vi "Set default remote state.vi"(8 "error in (no error)":errorcluster, 10 "Default remote state (Local)":u16(ring) items=["Local", "Remote"], 11 "VISA resource name":refnum<visa-resource-name>) -> (0 "error out":errorcluster, 3 "VISA resource name out":refnum<visa-resource-name>)   [LabVIEW 2020, in "Datron D4xxx.lvlib"]
doc: "This function does not affect GPIB REN state, it just sets its default value to which REN line is set after any command from this library or if you use \"Set remote state\" VI with default parameter."
uses:
  Datron D4xxx.lvlib
  Private/vars.vi
panel:
  out "VISA ID":i32
  # "Just some work variables"
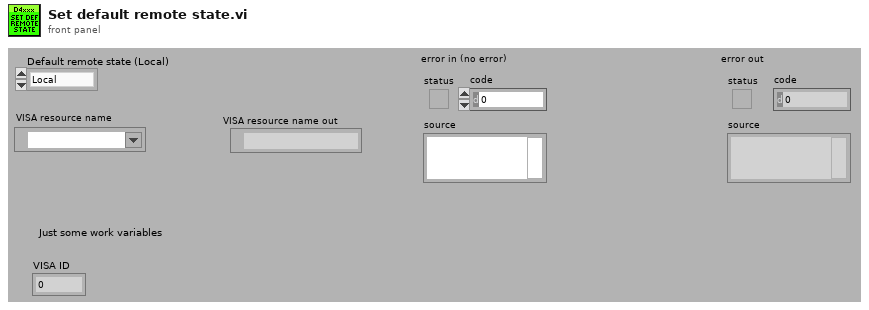
[diagram p1: front panel]
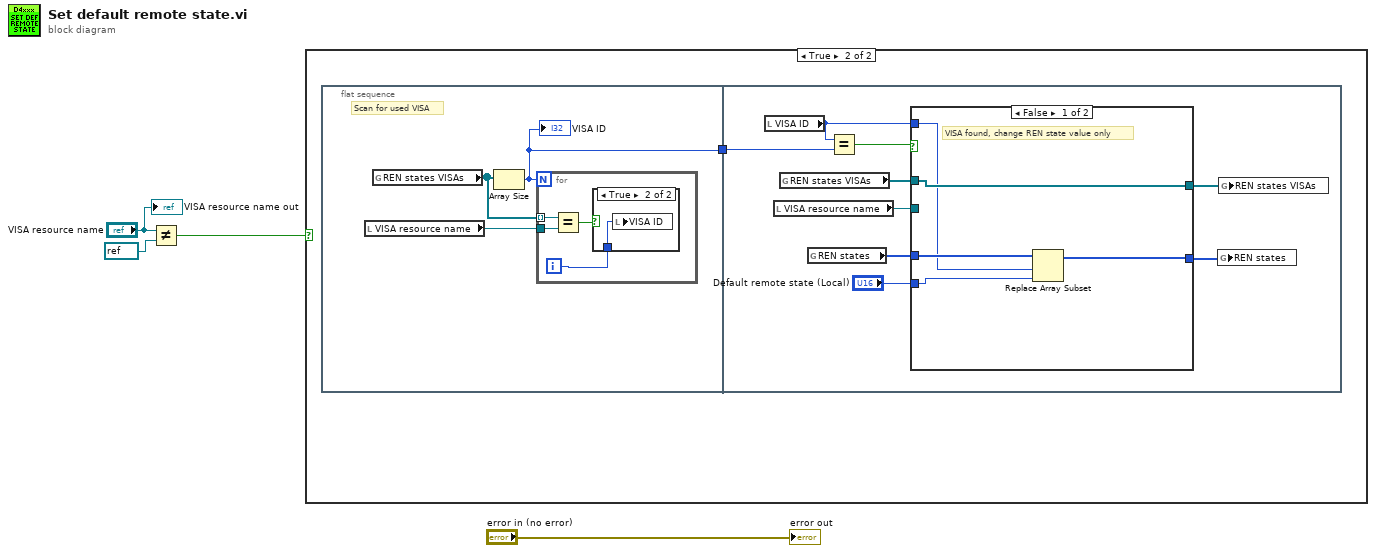
[diagram p0: block diagram]
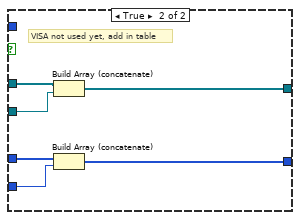
[diagram p4: hidden frame]
diagram:
  n1 = Not Equal?(x="VISA resource name", y=refnum<visa-resource-name> refnum ("VISA resource name out")) -> (x != y?=w2:bool)
  n2 = case shown="True" w2 {
    frame False {
    }
    frame True {
      n3 = flat-sequence {
        tunnel: [w7] -> w5
        tunnel: w5 -> [w15]
        frame #0 {
          # "Scan for used VISA"
          n4 = local read "VISA resource name"() -> (w6:refnum<visa-resource-name>)
          n5 = global read "vars.vi" "REN states VISAs"() -> (w8:refnum<visa-resource-name>[])
          n6 = Array Size(array=w8) -> (size(s)=w7:i32)
          "VISA ID" <- w7
          n7 = for {
            N: w7 -> [_]
            tunnel: w6 -> [w12]
            tunnel: w8 -> [w11] mode=indexing
            i -> [w9]
            n8 = Equal?(x=w11, y=w12) -> (x = y?=w10:bool)
            n9 = case shown="True" w10 {
              tunnel: w9 -> [_ w13]
              frame False {
              }
              frame True {
                n10 = local write "VISA ID"(w13) -> ()
              }
            }
          }
        }
        frame #1 {
          n11 = local read "VISA ID"() -> (w14:i32)
          n12 = local read "VISA resource name"() -> (w20:refnum<visa-resource-name>)
          n13 = global read "vars.vi" "REN states VISAs"() -> (w21:refnum<visa-resource-name>[])
          n14 = global read "vars.vi" "REN states"() -> (w18:u16[])
          n15 = Equal?(x=w14, y=w15) -> (x = y?=w22:bool)
          n16 = case shown="False" w22 {
            tunnel: w21 -> [w27 w33]
            tunnel: w20 -> [_ w32]
            tunnel: [w27 w31] -> w19
            tunnel: w18 -> [w26 w30]
            tunnel: "Default remote state (Local)" -> [w24 w29]
            tunnel: [w25 w28] -> w16
            tunnel: w14 -> [w23 _]
            frame False {
              # "VISA found, change REN state value only"
              n17 = Replace Array Subset(array=w26, new element=w24, index=w23) -> (w25:u16[])
            }
            frame True {
              # "VISA not used yet, add in table"
              n18 = Build Array (concatenate)(w33, w32) -> (w31:refnum<visa-resource-name>[])
              n19 = Build Array (concatenate)(w30, w29) -> (w28:u16[])
            }
          }
          n20 = global write "vars.vi" "REN states"(w16) -> ()
          n21 = global write "vars.vi" "REN states VISAs"(w19) -> ()
        }
      }
    }
  }
  "VISA resource name out" <- "VISA resource name"
  "error out" <- "error in (no error)"
